vi "加法范围自动适配大.vi"() -> ()   [LabVIEW 2020]
panel:
  out "U8":u8
  out "U8":u8
  out "数值":dbl
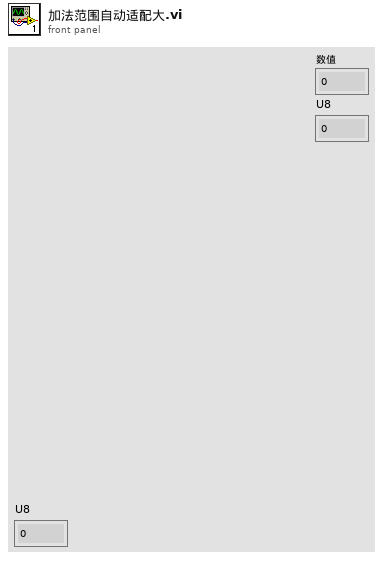
[diagram p1: front panel]
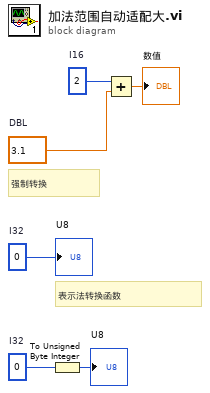
[diagram p0: block diagram]
diagram:
  w2 = 0  # I32
  w3 = 0  # I32
  w5 = 3.1  # DBL
  w6 = 2  # I16
  # "强制转换"
  # "表示法转换函数"
  n1 = To Unsigned Byte Integer(number=w2) -> (unsigned 8bit integer=→"U8":u8)
  n2 = Add(x=w6, y=w5) -> (x+y=→"数值":dbl)
  "U8" <- w3
